vi "Pins Disabled Write.vi"(4 "error in (no error)":errorcluster, 5 "Value":T1(array[ring]), 6 "Container State":T3, 7 "Display State In":T2) -> (0 "error out":errorcluster, 3 "Display State Out":T2)   [LabVIEW 2021, in "roboRIO 4 Bank.xctl"]
uses:
  <vilib>/myRIO/Common/Instrument Driver Framework/Utilities/xctls/roboRIO 4 Bank/roboRIO 4 Bank.xctl
  <vilib>/_xctls/Container State.ctl
  <vilib>/myRIO/Common/Instrument Driver Framework/Utilities/xctls/roboRIO 4 Bank/State.ctl
  <vilib>/myRIO/Common/Instrument Driver Framework/Utilities/xctls/utilities/vis/myRIOXC Error Strings Global.vi
  <vilib>/_xctls/XControlSupport.lvlib
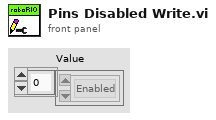
[diagram p1: front panel]
types:
  T1 = enum8{"Enabled", "Disabled", "Disabled and Grayed Out"}[]
  T2 = typedef "roboRIO 4 Bank.xctl/State.ctl" = cluster{"Pin Disabled?":enum8{"Enabled", "Disabled", "Disabled and Grayed Out"}[], "Pin Name":string[], "Pin ID":string[], "Connector Name":string, "Row Name 1":string, "Row Name 2":string}
  T3 = typedef "XControlSupport.lvlib/Container State.ctl" = cluster{"Indicator?":bool, "Run Mode?":bool, " Refnum":refnum<vi>}
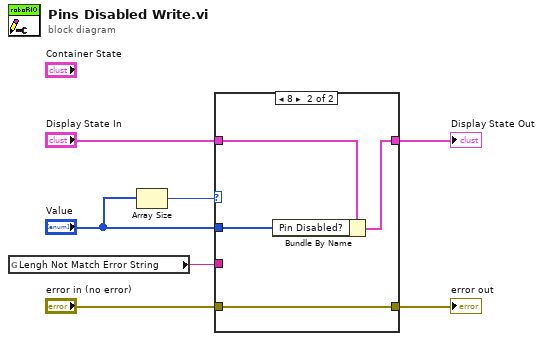
[diagram p0: block diagram]
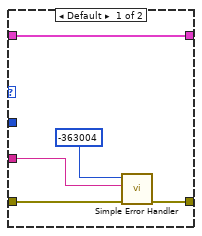
[diagram p2: hidden frame]
diagram:
  n1 = global read "myRIOXC Error Strings Global.vi" "Lengh Not Match Error String"() -> (w1:string)
  n2 = Array Size(array="Value") -> (size(s)=w7:i32)
  n3 = case shown="8" w7 {
    tunnel: "Value" -> [_ w15]
    tunnel: "Display State In" -> [w10 w16]
    tunnel: [w10 w14] -> w2
    tunnel: w1 -> [w8 _]
    tunnel: "error in (no error)" -> [w12 w13]
    tunnel: [w11 w13] -> w3
    frame Default {
      n4 = call <vilib>:"Simple Error Handler.vi"("error code (no error:0)"=-363004, "error source (\" \")"=w8, "error in (no error)"=w12) -> ("error out"=w11:errorcluster)  [unwired: 2 in, 4 out]
    }
    frame 8 {
      n5 = Bundle By Name(cluster=w16, "Pin Disabled?"=w15) -> (w14:T2)
    }
  }
  "error out" <- w3
  "Display State Out" <- w2
